vi "ERA_SS_Estimation.vi"(7 "Order Index":i32, 8 "Error In":errorcluster, 10 "H_1":T1, 11 "H_0":T1) -> (0 "Error Out":errorcluster, 2 "A":T1, 4 "C":T1, 6 "B":T1)   [LabVIEW 2017, in "AppPlugins.lvlib" / "EraPlugin.lvclass"]
uses:
  EraPlugin.lvclass
  <vilib>/Analysis/Matrix/Datatypes/RealMatrix.ctl
  <vilib>/Analysis/7linalg.llb/SVD Option.ctl
  <vilib>/Analysis/baseanly.llb/Real A x B.vi
  <vilib>/Analysis/7linalg.llb/Real SVD Decomposition.vi
  <vilib>/Analysis/7linalg.llb/Create Special Real Matrix.vi
  <vilib>/Analysis/NI_AALBase.lvlib
  <vilib>/Analysis/NI_AALPro.lvlib
  <vilib>/Analysis/Matrix/NI_Matrix.lvlib
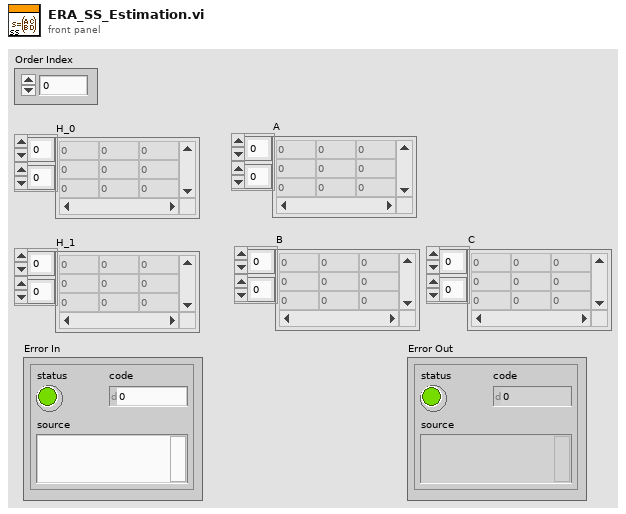
[diagram p1: front panel]
types:
  T1 = typedef "NI_Matrix.lvlib/RealMatrix.ctl" = dbl[][]
  T2 = typedef "NI_AALPro.lvlib/SVD Option.ctl" = u16
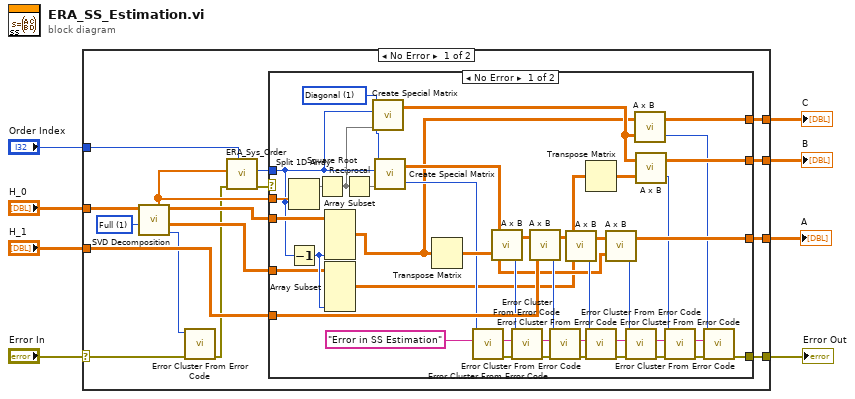
[diagram p0: block diagram]
diagram:
  n1 = case shown="No Error" "Error In" {
    selector: "Error In" -> [w13 w63]
    tunnel: "H_1" -> [w24 _]
    tunnel: "H_0" -> [w23 _]
    tunnel: [w22 _] -> w6
    tunnel: "Order Index" -> [w17 _]
    tunnel: [w15 w63] -> w4
    tunnel: [w10 _] -> w2
    tunnel: [w9 _] -> w1
    frame No Error {
      w14 = T2 1 items=["Thin", "Full"] ("SVD option")
      n2 = call-poly <vilib>:"SVD Decomposition.vi"("SVD option"=w14, "A"=w23) -> ("error"=w11:i32, "Matrix V"=w20:T1, "Matrix U"=w19:T1, "Vector S"=w21:dbl[])  [unwired: 5 in, 1 out]
      n3 = call <vilib>:"Error Cluster From Error Code.vi"("error in (no error)"=w13, "error code (0)"=w11) -> ("error out"=w12:errorcluster)  [unwired: 7 in]
      n4 = call "ERA_Sys_Order.vi"("Threshold"=w17, "Error In"=w12, "Vector S"=w21) -> ("Error Out"=w16:errorcluster, "System Order"=w18:i32)  [unwired: 7 in]
      n5 = case shown="No Error" w16 {
        selector: w16 -> [_ w62]
        tunnel: w24 -> [w59 _]
        tunnel: [w58 _] -> w22
        tunnel: w21 -> [w54 _]
        tunnel: w20 -> [w53 _]
        tunnel: w19 -> [w52 _]
        tunnel: w18 -> [w39 _]
        tunnel: [w28 w62] -> w15
        tunnel: [w36 _] -> w10
        tunnel: [w35 _] -> w9
        frame No Error {
          w25 = "Error in SS Estimation" ("error message (\"\")")
          w38 = 1 items=["Identity", "Diagonal", "Toeplitz", "Vandermonde", "Companion", "Hankel", "Hadamard", "Wilkinson", "Hilbert", "Inverse Hilbert", "Rosser", "Pascal"] ("matrix type")
          n6 = Split 1D Array(array=w54, index=w39) -> (first subarray=w41:dbl[])  [unwired: 1 out]
          n7 = Decrement(x=w39) -> (x-1=w61:i32)
          n8 = Square Root(x=w41) -> (sqrt(x)=w37:dbl[])
          n9 = Array Subset(array=w52, length (col)=w61) -> (w33:T1)  [unwired: 3 in]
          n10 = Array Subset(array=w53, length (col)=w61) -> (w31:T1)  [unwired: 3 in]
          n11 = Reciprocal(x=w37) -> (1/x=w40:dbl[])
          n12 = call-poly <vilib>:"Create Special Matrix.vi"("matrix type"=w38, "matrix size"=w39, "Input Vector1"=w37) -> ("Special Matrix"=w34:T1)  [unwired: 2 in, 1 out]
          n13 = call-poly <vilib>:"Create Special Matrix.vi"("matrix type"=w38, "matrix size"=w39, "Input Vector1"=w40) -> ("Special Matrix"=w42:T1, "error"=w51:i32)  [unwired: 2 in]
          n14 = Transpose Matrix(1:w33) -> (0:w60:T1)
          n15 = call <vilib>:"Error Cluster From Error Code.vi"("error message (\"\")"=w25, "error code (0)"=w51) -> ("error out"=w50:errorcluster)  [unwired: 7 in]
          n16 = call-poly <vilib>:"A x B.vi"("B"=w60, "A"=w42) -> ("error"=w46:i32, "A x B"=w56:T1)
          n17 = call <vilib>:"Error Cluster From Error Code.vi"("error in (no error)"=w50, "error message (\"\")"=w25, "error code (0)"=w46) -> ("error out"=w49:errorcluster)  [unwired: 6 in]
          n18 = call-poly <vilib>:"A x B.vi"("B"=w59, "A"=w56) -> ("error"=w45:i32, "A x B"=w57:T1)
          n19 = call <vilib>:"Error Cluster From Error Code.vi"("error in (no error)"=w49, "error message (\"\")"=w25, "error code (0)"=w45) -> ("error out"=w48:errorcluster)  [unwired: 6 in]
          n20 = call-poly <vilib>:"A x B.vi"("B"=w31, "A"=w57) -> ("error"=w44:i32, "A x B"=w55:T1)
          n21 = Transpose Matrix(1:w31) -> (0:w32:T1)
          n22 = call <vilib>:"Error Cluster From Error Code.vi"("error in (no error)"=w48, "error message (\"\")"=w25, "error code (0)"=w44) -> ("error out"=w47:errorcluster)  [unwired: 6 in]
          n23 = call-poly <vilib>:"A x B.vi"("B"=w42, "A"=w55) -> ("error"=w43:i32, "A x B"=w58:T1)
          n24 = call <vilib>:"Error Cluster From Error Code.vi"("error in (no error)"=w47, "error message (\"\")"=w25, "error code (0)"=w43) -> ("error out"=w30:errorcluster)  [unwired: 6 in]
          n25 = call-poly <vilib>:"A x B.vi"("B"=w34, "A"=w33) -> ("error"=w26:i32, "A x B"=w36:T1)
          n26 = call-poly <vilib>:"A x B.vi"("B"=w32, "A"=w34) -> ("error"=w27:i32, "A x B"=w35:T1)
          n27 = call <vilib>:"Error Cluster From Error Code.vi"("error in (no error)"=w30, "error message (\"\")"=w25, "error code (0)"=w27) -> ("error out"=w29:errorcluster)  [unwired: 6 in]
          n28 = call <vilib>:"Error Cluster From Error Code.vi"("error in (no error)"=w29, "error message (\"\")"=w25, "error code (0)"=w26) -> ("error out"=w28:errorcluster)  [unwired: 6 in]
        }
        frame Error {
        }
      }
    }
    frame Error {
    }
  }
  "A" <- w6
  "Error Out" <- w4
  "C" <- w2
  "B" <- w1
